vi "Game Data.vi"(3 "error in":errorcluster) -> (1 "Game Specific Data":string)   [LabVIEW 2017]
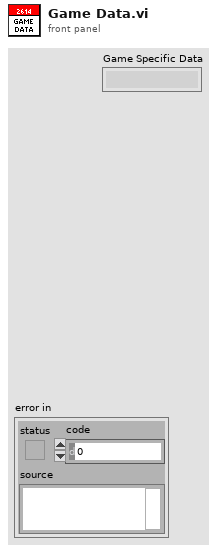
[diagram p1: front panel]
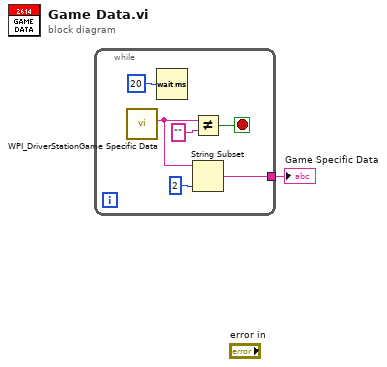
[diagram p0: block diagram]
diagram:
  n1 = while {
    tunnel: [w2] -> w1
    stop <- w6 stop-if-true
    n2 = call <vilib>:"WPI_DriverStationGame Specific Data.vi"() -> ("Game Specific Data"=w3:string)  [unwired: 11 in]
    n3 = Wait (ms)(milliseconds to wait=u32 20) -> ()  [unwired: 1 out]
    n4 = Not Equal?(x=w3, y="") -> (x != y?=w6:bool)
    n5 = String Subset(string=w3, length (rest)=2 ("length (rest)")) -> (substring=w2:string)  [unwired: 1 in]
  }
  "Game Specific Data" <- w1
